vi "FA_BuildPath.vi"(7 "LSCollections":T2, 8 "error in (no error)":errorcluster, 9 "Item Name":string, 10 "Special Type":T1, 11 "FlockAgentLocalStore":path=path "c:/FlockAgentLocalStore") -> (0 "error out":errorcluster, 2 "directory path":path, 3 "file path":path)   [LabVIEW 2014, in "FA_LocalStore.lvlib"]
doc: "Given a Special Type this VI returns the location within LocalStore of that Special Types data. If a directory for a given Special Type does not exist, this VI will create it. This VI defaults the LocalStore location to C:\\FlockAgentLocalStore\\ but any relative path can be used by passing a path to the FlockAgentLocalStore input. \n\nIf the value for LSCollections is Config Item and no Item Name is specified the VI returns items.xml for the file path for a particular special type. If an Item Name is specific the VI returns the item path."
uses:
  FA_LocalStore.lvlib
  FA_LSCollections.ctl
  FA_LSSpecialTypes.ctl
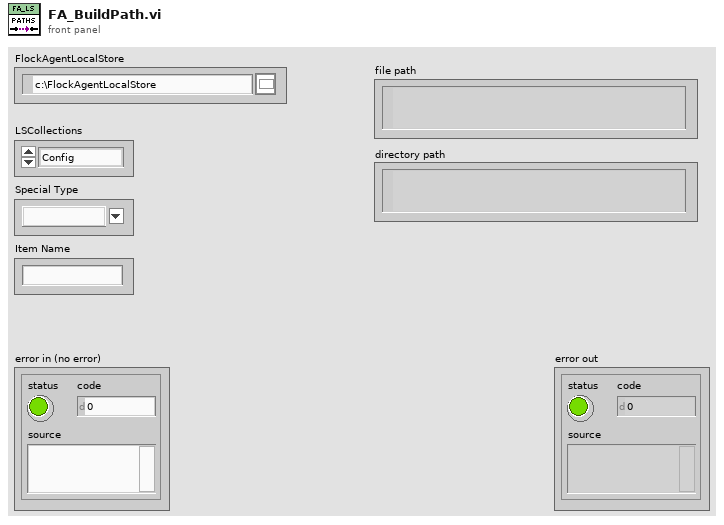
[diagram p1: front panel]
types:
  T1 = typedef "FA_LocalStore.lvlib/FA_LSSpecialTypes.ctl" = string
  T2 = typedef "FA_LocalStore.lvlib/FA_LSCollections.ctl" = enum16{"Config", "ConfigItem", "FA_eTag", "FA_PlugIn"}
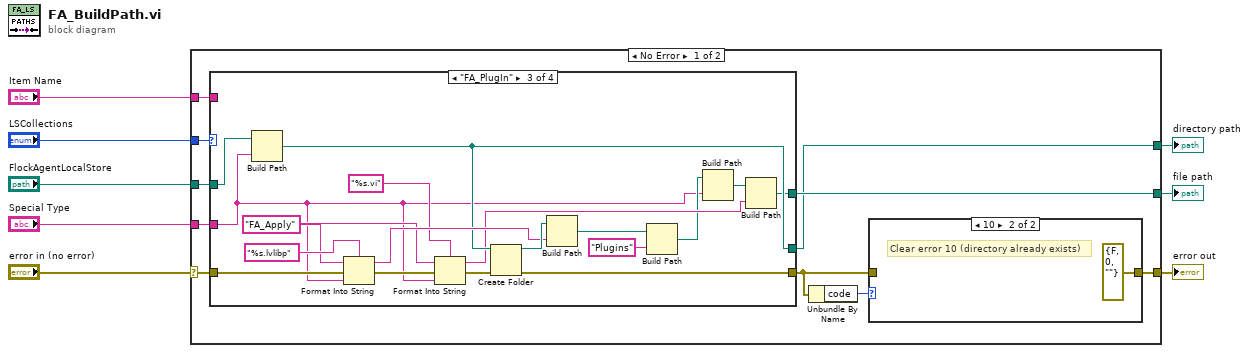
[diagram p0: block diagram]
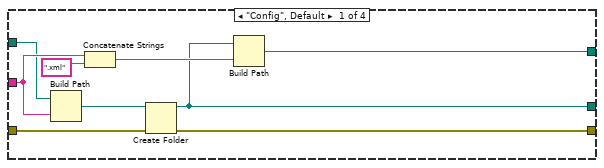
[diagram p3: hidden frame]
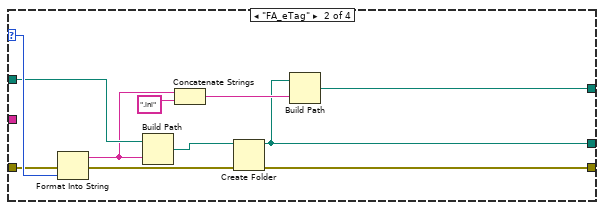
[diagram p4: hidden frame]
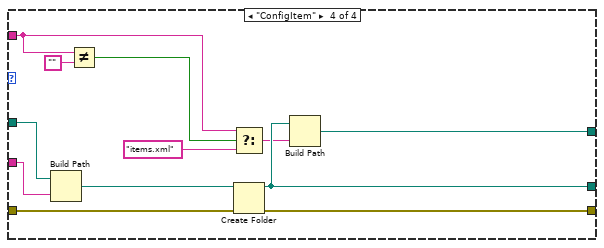
[diagram p5: hidden frame]
diagram:
  n1 = case shown="No Error" "error in (no error)" {
    selector: "error in (no error)" -> [w12 w71]
    tunnel: [w14 w71] -> w5
    tunnel: "Special Type" -> [w17 _]
    tunnel: "FlockAgentLocalStore" -> [w16 _]
    tunnel: "LSCollections" -> [w15 _]
    tunnel: [w13 _] -> w4
    tunnel: [w10 _] -> w2
    tunnel: "Item Name" -> [w9 _]
    frame No Error {
      n2 = case shown="\"FA_PlugIn\"" w15 {
        selector: w15 -> [_ w37 _ _]
        tunnel: w17 -> [w27 _ w41 w64]
        tunnel: [w25 w32 w51 w68] -> w13
        tunnel: [w24 w35 w52 w66] -> w11
        tunnel: w16 -> [w23 w34 w57 w69]
        tunnel: w12 -> [w21 w31 w53 w67]
        tunnel: [w22 w30 w54 w65] -> w10
        tunnel: w9 -> [_ _ _ w61]
        frame "Config", Default {
          n3 = Build Path(base path=w23, name or relative path=w27) -> (appended path=w29:path)
          n4 = Concatenate Strings(w27, ".xml" ("string")) -> (w26:string)
          n5 = Create Folder(path (use dialog)=w29, error in=w21) -> (created path=w22:path, error out=w24:errorcluster)  [unwired: 1 in, 1 out]
          n6 = Build Path(base path=w22, name or relative path=w26) -> (appended path=w25:path)
        }
        frame "FA_eTag" {
          n7 = Format Into String(error in=w31, w37) -> (resulting string=w33:string, error out=w36:errorcluster)  [unwired: 2 in]
          n8 = Build Path(base path=w34, name or relative path=w33) -> (appended path=w38:path)
          n9 = Concatenate Strings(w33, ".ini" ("name or relative path")) -> (w40:string)
          n10 = Create Folder(path (use dialog)=w38, error in=w36) -> (created path=w30:path, error out=w35:errorcluster)  [unwired: 1 in, 1 out]
          n11 = Build Path(base path=w30, name or relative path=w40) -> (appended path=w32:path)
        }
        frame "FA_PlugIn" {
          w49 = "FA_Apply" ("initial string")
          n12 = Build Path(base path=w57, name or relative path=w41) -> (appended path=w54:path)
          n13 = Format Into String(format string="%s.lvlibp", initial string=w49, error in=w53, w41) -> (resulting string=w55:string, error out=w48:errorcluster)
          n14 = Format Into String(format string="%s.vi", initial string=w49, error in=w48, w41) -> (resulting string=w45:string, error out=w47:errorcluster)
          n15 = Create Folder(path (use dialog)=w54, error in=w47) -> (created path=w58:path, error out=w52:errorcluster)  [unwired: 1 in, 1 out]
          n16 = Build Path(base path=w58, name or relative path=w55) -> (appended path=w46:path)
          n17 = Build Path(base path=w46, name or relative path="Plugins") -> (appended path=w44:path)
          n18 = Build Path(base path=w44, name or relative path=w41) -> (appended path=w42:path)
          n19 = Build Path(base path=w42, name or relative path=w45) -> (appended path=w51:path)
        }
        frame "ConfigItem" {
          n20 = Build Path(base path=w69, name or relative path=w64) -> (appended path=w70:path)
          n21 = Not Equal?(x=w61, y="") -> (x != y?=w62:bool)
          n22 = Select(t=w61, s=w62, f="items.xml") -> (s? t:f=w59:string)
          n23 = Create Folder(path (use dialog)=w70, error in=w67) -> (created path=w65:path, error out=w66:errorcluster)  [unwired: 1 in, 1 out]
          n24 = Build Path(base path=w65, name or relative path=w59) -> (appended path=w68:path)
        }
      }
      n25 = Unbundle By Name(w11) -> ("code"=w18:i32)
      n26 = case shown="10" w18 {
        tunnel: [w19 errorcluster {"status"=FALSE, "code"=0, "source"=""} ("error IO")] -> w14
        tunnel: w11 -> [w19 _]
        frame 0, Default {
        }
        frame 10 {
          # "Clear error 10 (directory already exists)"
        }
      }
    }
    frame Error {
    }
  }
  "file path" <- w4
  "error out" <- w5
  "directory path" <- w2
